vi "RobotDriveMecanumUpdateSRXSpeed.vi"(6 "Rear Right":dbl, 7 "Rear Left":dbl, 8 "error in":errorcluster, 9 "Front Right":dbl, 10 "Front Left":dbl, 11 "RobotDriveDevRef in":T2) -> (0 "error out":errorcluster, 1 "SRX Status":T1[](array[typedef]), 2 "Motor Values":dbl[](array[numeric]), 3 "RobotDriveDevRef out":T2)   [LabVIEW 2016]
uses:
  <vilib>/Rock Robotics/WPI/RobotDrive/WPI_RobotDriveDevRef.ctl
  <vilib>/Rock Robotics/WPI/MotorControl/WPI_MotorControlDeviceRef.ctl
  <vilib>/Rock Robotics/WPI/MotorControl/WPI_MotorControlType.ctl
  <vilib>/Rock Robotics/SystemInterfaces/DIO/FPGA_DIOPWMChannel.ctl
  <vilib>/Rock Robotics/WPI/PWM/WPI_PWMDeadband.ctl
  <vilib>/Rock Robotics/WPI/ThirdParty/CanMotor/TalonSRX/WPI_CANTalonSRX_GlobalStatus.ctl
  <vilib>/Rock Robotics/WPI/RobotDrive/WPI_RobotDriveMotorSelectorEnum.ctl
  <vilib>/Rock Robotics/WPI/RobotDrive/WPI_RobotDriveSafetyCheck.vi
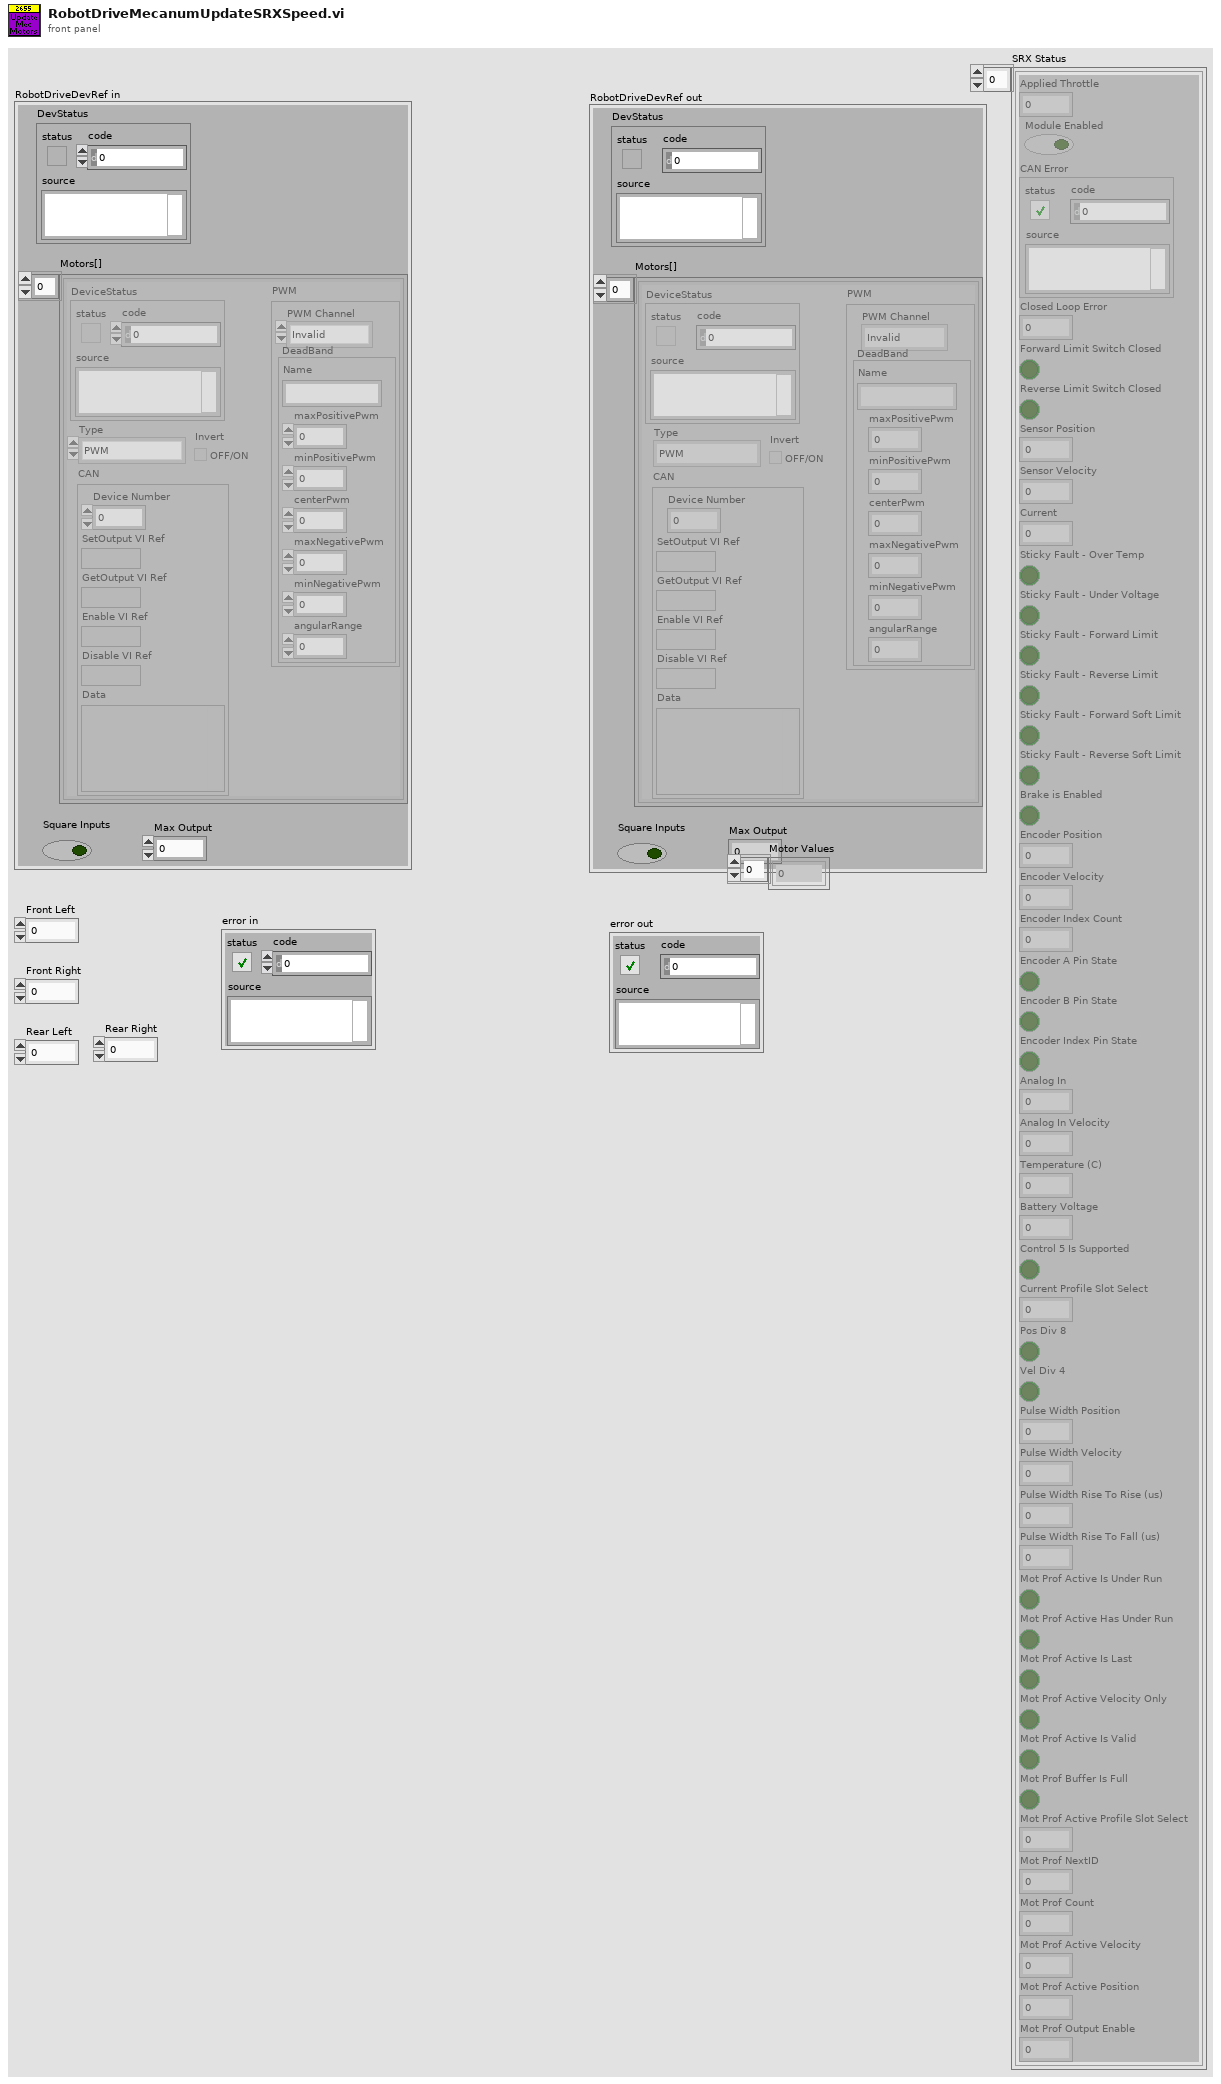
[diagram p1: front panel]
types:
  T1 = typedef "WPI_CANTalonSRX_GlobalStatus.ctl" = cluster{"Applied Throttle":dbl, "Module Enabled":bool, "CAN Error":errorcluster, "Closed Loop Error":dbl, "Forward Limit Switch Closed":bool, "Reverse Limit Switch Closed":bool, "Sensor Position":dbl, "Sensor Velocity":dbl, "Current":dbl, "Sticky Fault - Over Temp":bool, "Sticky Fault - Under Voltage":bool, "Sticky Fault - Forward Limit":bool, "Sticky Fault - Reverse Limit":bool, "Sticky Fault - Forward Soft Limit":bool, "Sticky Fault - Reverse Soft Limit":bool, "Brake is Enabled":bool, "Encoder Position":dbl, "Encoder Velocity":dbl, "Encoder Index Count":dbl, "Encoder A Pin State":bool, "Encoder B Pin State":bool, "Encoder Index Pin State":bool, "Analog In":dbl, "Analog In Velocity":dbl, "Temperature (C)":dbl, "Battery Voltage":dbl, "Control 5 Is Supported":bool, "Current Profile Slot Select":dbl, "Pos Div 8":bool, "Vel Div 4":bool, "Pulse Width Position":i32, "Pulse Width Velocity":i32, "Pulse Width Rise To Rise (us)":i32, "Pulse Width Rise To Fall (us)":i32, "Mot Prof Active Is Under Run":bool, "Mot Prof Active Has Under Run":bool, "Mot Prof Active Is Last":bool, "Mot Prof Active Velocity Only":bool, "Mot Prof Active Is Valid":bool, "Mot Prof Buffer Is Full":bool, "Mot Prof Active Profile Slot Select":i32, "Mot Prof NextID":i32, "Mot Prof Count":i32, "Mot Prof Active Velocity":dbl, "Mot Prof Active Position":dbl, "Mot Prof Output Enable":i32}
  T2 = typedef "WPI_RobotDriveDevRef.ctl" = cluster{"DevStatus":errorcluster, "Motors[]":T3[], "Square Inputs":bool, "Max Output":dbl}
  T3 = typedef "WPI_MotorControlDeviceRef.ctl" = cluster{"DeviceStatus":errorcluster, "Type":T4, "PWM":cluster{"PWM Channel":T5, "DeadBand":T6}, "CAN":cluster{"Device Number":u8, "SetOutput VI Ref":variant, "GetOutput VI Ref":variant, "Enable VI Ref":variant, "Disable VI Ref":variant, "Data":variant}, "Invert":bool}
  T4 = typedef "WPI_MotorControlType.ctl" = enum16{"PWM", "CAN"}
  T5 = typedef "FPGA_DIOPWMChannel.ctl" = enum8{"PWM 0", "PWM 1", "PWM 2", "PWM 3", "PWM 4", "PWM 5", "PWM 6", "PWM 7", "PWM 8", "PWM 9", "PWM MXP 0", "PWM MXP 1", "PWM MXP 2", "PWM MXP 3", "PWM MXP 4", "PWM MXP 5", "PWM MXP 6", "PWM MXP 7", "PWM MXP 8", "PWM MXP 9", "Invalid"}
  T6 = typedef "WPI_PWMDeadband.ctl" = cluster{"Name":string, "maxPositivePwm":i32, "minPositivePwm":i32, "centerPwm":i32, "maxNegativePwm":i32, "minNegativePwm":i32, "angularRange":u16}
  T7 = typedef "WPI_RobotDriveMotorSelectorEnum.ctl" = enum16{"Rear Left Motor", "Rear Right Motor", "Front Left Motor", "Front Right Motor"}
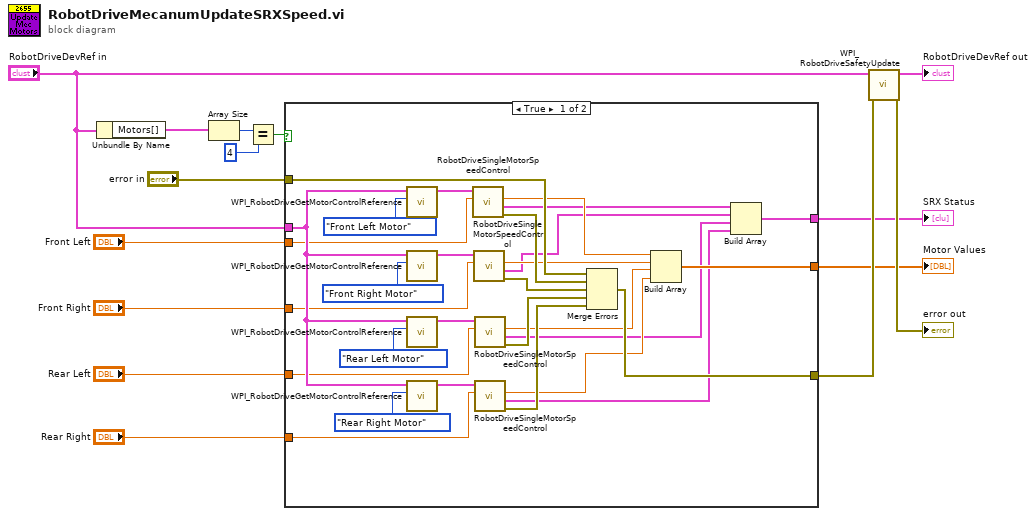
[diagram p0: block diagram]
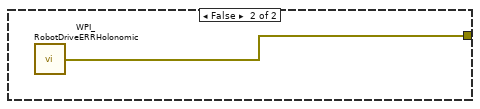
[diagram p2: hidden frame]
diagram:
  n1 = Unbundle By Name("RobotDriveDevRef in") -> ("Motors[]"=w8:T3[])
  n2 = Array Size(array=w8) -> (size(s)=w4:i32)
  n3 = Equal?(x=w4, y=4) -> (x = y?=w6:bool)
  n4 = case shown="True" w6 {
    tunnel: "Front Left" -> [w25 _]
    tunnel: "Front Right" -> [w26 _]
    tunnel: "RobotDriveDevRef in" -> [w40 _]
    tunnel: [w39 w45] -> w7
    tunnel: "Rear Left" -> [w27 _]
    tunnel: "Rear Right" -> [w28 _]
    tunnel: [w38 _] -> w2
    tunnel: "error in" -> [w37 _]
    tunnel: [w16 _] -> w1
    frame True {
      n5 = call <vilib>:"WPI_RobotDriveGetMotorControlReference.vi"("MotorIndex"=WPI_RobotDriveMotorSelectorEnum."Front Left Motor", "RobotDriveDevRef"=w40) -> ("MotorControlDeviceRef"=w36:T3)  [unwired: 9 out]
      n6 = call <vilib>:"WPI_RobotDriveGetMotorControlReference.vi"("MotorIndex"=WPI_RobotDriveMotorSelectorEnum."Front Right Motor", "RobotDriveDevRef"=w40) -> ("MotorControlDeviceRef"=w33:T3)  [unwired: 9 out]
      n7 = call <vilib>:"WPI_RobotDriveGetMotorControlReference.vi"("MotorIndex"=WPI_RobotDriveMotorSelectorEnum."Rear Left Motor", "RobotDriveDevRef"=w40) -> ("MotorControlDeviceRef"=w32:T3)  [unwired: 9 out]
      n8 = call <vilib>:"WPI_RobotDriveGetMotorControlReference.vi"("MotorIndex"=WPI_RobotDriveMotorSelectorEnum."Rear Right Motor", "RobotDriveDevRef"=w40) -> ("MotorControlDeviceRef"=w30:T3)  [unwired: 9 out]
      n9 = call "RobotDriveSingleMotorSpeedControl.vi"("Joystick Input"=w25, "CAN Talon SRX Ref"=w36) -> ("error out"=w35:errorcluster, "Talon SRX Status"=w20:T1, "Target RPM"=w24:dbl)  [unwired: 7 in]
      n10 = call "RobotDriveSingleMotorSpeedControl.vi"("Joystick Input"=w26, "CAN Talon SRX Ref"=w33) -> ("error out"=w34:errorcluster, "Talon SRX Status"=w19:T1, "Target RPM"=w23:dbl)  [unwired: 7 in]
      n11 = call "RobotDriveSingleMotorSpeedControl.vi"("Joystick Input"=w27, "CAN Talon SRX Ref"=w32) -> ("error out"=w31:errorcluster, "Talon SRX Status"=w18:T1, "Target RPM"=w22:dbl)  [unwired: 7 in]
      n12 = call "RobotDriveSingleMotorSpeedControl.vi"("Joystick Input"=w28, "CAN Talon SRX Ref"=w30) -> ("error out"=w29:errorcluster, "Talon SRX Status"=w17:T1, "Target RPM"=w21:dbl)  [unwired: 7 in]
      n13 = Merge Errors(w37, w35, w34, w31, w29) -> (w39:errorcluster)
      n14 = Build Array(w24, w23, w22, w21) -> (w38:dbl[])
      n15 = Build Array(w20, w19, w18, w17) -> (w16:T1[])
    }
    frame False {
      n16 = call <vilib>:"WPI_RobotDriveERRHolonomic.vi"() -> ("error out"=w45:errorcluster)
    }
  }
  "Motor Values" <- w2
  "SRX Status" <- w1
  n17 = call <vilib>:"WPI_RobotDriveSafetyUpdate.vi"("error in (no error)"=w7, "RobotDriveDevRef"="RobotDriveDevRef in") -> ("error out"=→"error out":errorcluster, "RobotDriveDevRef"=→"RobotDriveDevRef out":T2)  [unwired: 8 out]
